vi "Build Failure Action Menu.vi"(8 "error in (no error)":errorcluster, 10 "Assert VI UID":i32, 11 "Menu in":refnum<k9>) -> (0 "error out":errorcluster)   [LabVIEW 2016, in "Assert API Components.lvlib" / "Assert Display.lvlib" / "Main Display.lvlib" / "Main Display.lvclass"]
doc: "Builds up the failure action using the selected UID and adds in items for None, Log To File, Pause Execution and Abort Execution"
uses:
  Main Display.lvclass
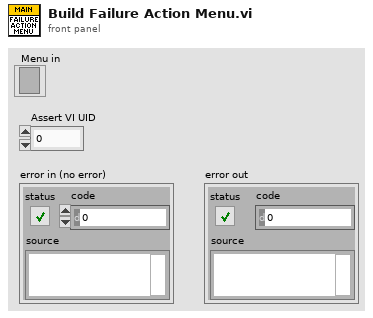
[diagram p1: front panel]
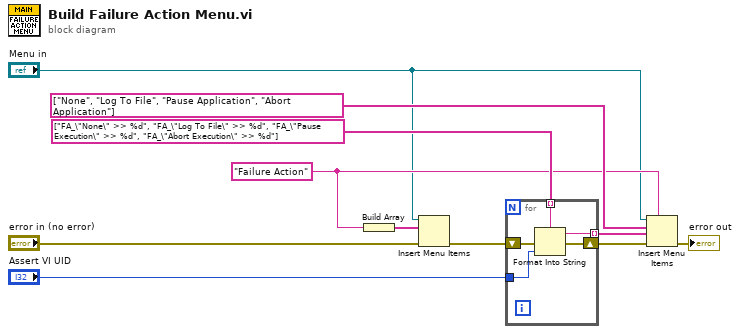
[diagram p0: block diagram]
diagram:
  w5 = "Failure Action"
  n1 = Build Array(w5) -> (w2:string[])
  n2 = Insert Menu Items(6:"error in (no error)", 8:w2, 9:"Menu in") -> (0:w1:errorcluster)  [unwired: 3 in, 2 out]
  n3 = for {
    tunnel: "Assert VI UID" -> [w15]
    shift-right: [w14] -> w8
    shift-left: w1 -> [w16]
    tunnel: string[] ["FA_\"None\" >> %d", "FA_\"Log To File\" >> %d", "FA_\"Pause Execution\" >> %d", "FA_\"Abort Execution\" >> %d"] -> [w13] mode=indexing
    tunnel: [w12] -> w10 mode=indexing
    n4 = Format Into String(format string=w13, error in=w16, w15) -> (resulting string=w12:string, error out=w14:errorcluster)  [unwired: 1 in]
  }
  n5 = Insert Menu Items(5:w5, 6:w8, 7:w10, 8:string[] ["None", "Log To File", "Pause Application", "Abort Application"], 9:"Menu in") -> (0:→"error out":errorcluster)  [unwired: 1 in, 2 out]
